vi "stimulus_sample_info.vi"(10 "Frequency":dbl, 11 "Length":dbl) -> (0 "Sample frequency":dbl, 1 "Actual frequency":dbl, 2 "Actual length":dbl, 3 "Num samples":i32)   [LabVIEW 2013]
panel:
  # "Discretize desired length and frequency according sampling frequency so that one or more whole cycles fit into the stimulus."
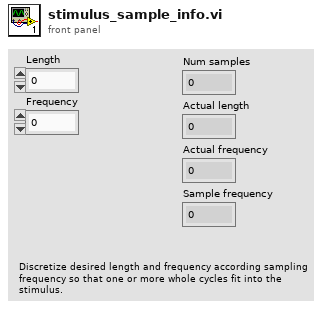
[diagram p1: front panel]
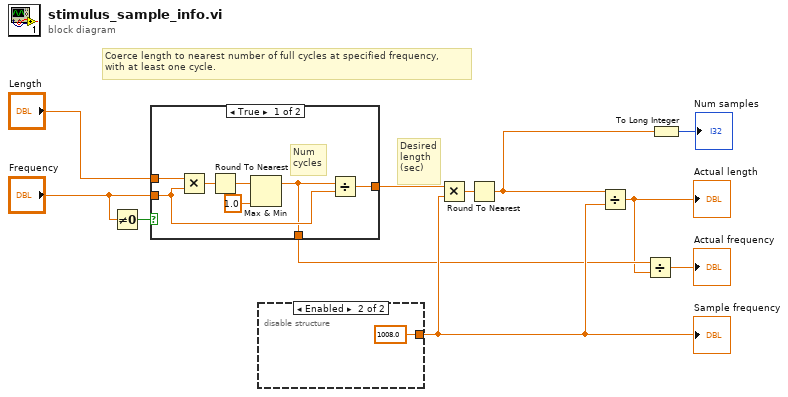
[diagram p0: block diagram]
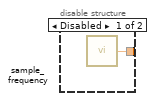
[diagram p2: hidden frame]
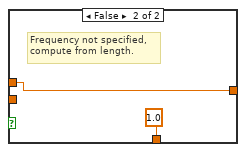
[diagram p3: hidden frame]
diagram:
  # "Desired\nlength\n(sec)"
  # "Coerce length to nearest number of full cycles at specified frequency,\nwith at least one cycle."
  n1 = Not Equal To 0?(x="Frequency") -> (x != 0?=w3:bool)
  n2 = case shown="True" w3 {
    tunnel: "Length" -> [w18 w20]
    tunnel: "Frequency" -> [w17 _]
    tunnel: [w13 1.0] -> w10
    tunnel: [w12 w20] -> w1
    frame True {
      # "Num \ncycles"
      n3 = Multiply(x=w18, y=w17) -> (x*y=w16:dbl)
      n4 = Round To Nearest(number=w16) -> (nearest integer value=w15:dbl)
      n5 = Max & Min(x=w15, y=1.0) -> (max(x,y)=w13:dbl)  [unwired: 1 out]
      n6 = Divide(x=w13, y=w17) -> (x/y=w12:dbl)
    }
    frame False {
      # "Frequency not specified,\ncompute from length."
    }
  }
  n7 = disable-structure shown="Enabled" {
    disable-tunnel: [w21 1008.0 ("Sample frequency")] -> w11
    frame Disabled {
      n8 = call "sample_frequency.vi"() -> ("Sample frequency"=w21:dbl)
    }
    frame Enabled {
    }
  }
  "Sample frequency" <- w11
  n9 = Multiply(x=w1, y=w11) -> (x*y=w2:dbl)
  n10 = Round To Nearest(number=w2) -> (nearest integer value=w7:dbl)
  n11 = Divide(x=w7, y=w11) -> (x/y=w9:dbl)
  "Actual length" <- w9
  n12 = Divide(x=w10, y=w9) -> (x/y=→"Actual frequency":dbl)
  n13 = To Long Integer(number=w7) -> (32bit integer=→"Num samples":i32)
